vi "MagX Probes to Listbox.vi"(8 "error in":errorcluster, 10 "Probes":T1[](array[typedef]), 11 "Listbox ref":refnum<vi>) -> (0 "error out":errorcluster, 3 "Listbox ref out":refnum<vi>)   [LabVIEW 2024]
uses:
  Probe info.ctl
panel:
  out "Listbox out":i32(listbox)
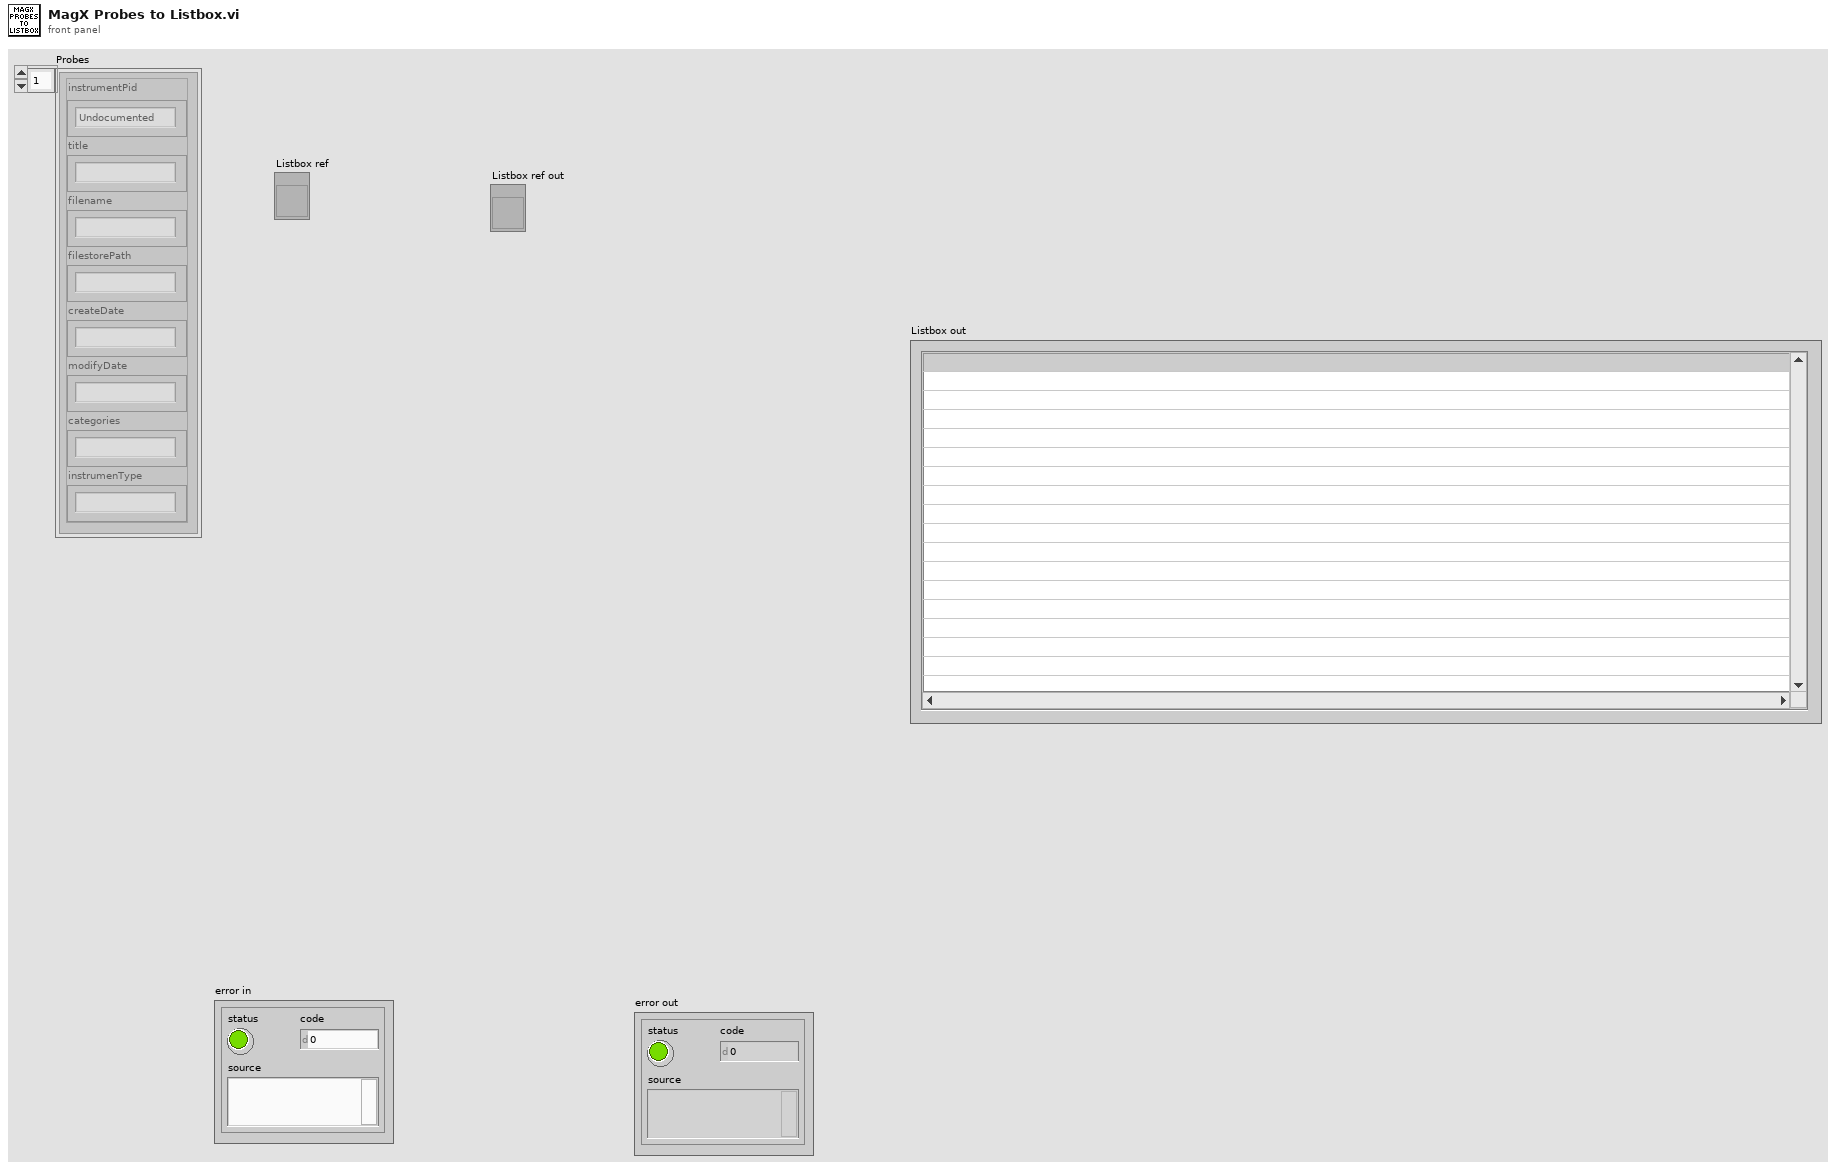
[diagram p1: front panel]
types:
  T1 = typedef "Probe info.ctl" = cluster{"instrumentPid":string, "title":string, "filename":string, "filestorePath":string, "createDate":string, "modifyDate":string, "categories":string, "instrumenType":string}
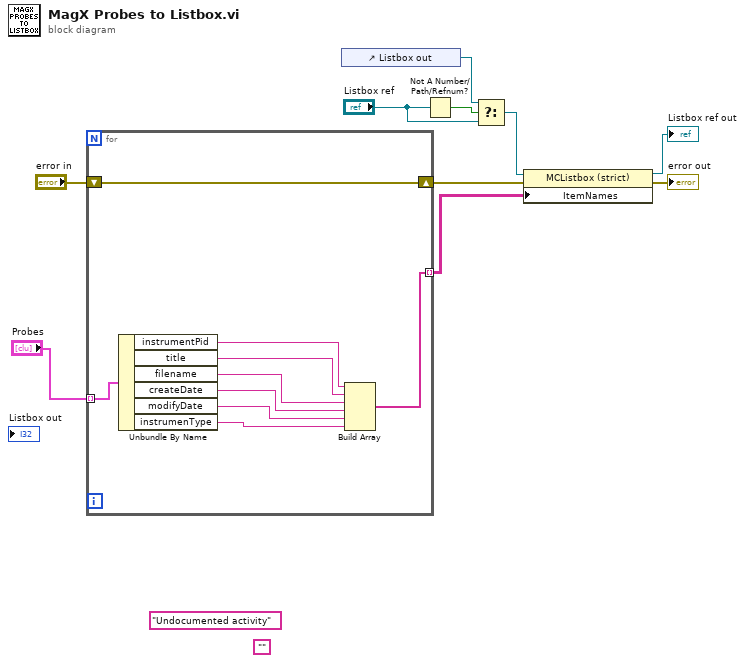
[diagram p0: block diagram]
diagram:
  (unwired) ""
  (unwired) "Undocumented activity"
  n1 = for {
    shift-right: [w19] -> w7
    shift-left: "error in" -> [w19]
    tunnel: [w11] -> w6 mode=indexing
    tunnel: "Probes" -> [w18] mode=indexing
    n2 = Unbundle By Name(w18) -> ("instrumentPid"=w17:string, "title"=w16:string, "filename"=w15:string, "createDate"=w14:string, "modifyDate"=w13:string, "instrumenType"=w12:string)
    n3 = Build Array(w17, w16, w15, w14, w13, w12) -> (w11:string[])
  }
  n4 = control-ref of="Listbox out"() -> (w4:refnum<vi>)
  n5 = Not A Number/Path/Refnum?(number/path/refnum="Listbox ref") -> (NaN/Path/Refnum?=w5:bool)
  n6 = Select(t=w4, s=w5, f="Listbox ref") -> (s? t:f=w2:refnum<vi>)
  n7 = property class="MCListbox (strict)"(reference=w2, error in=w7, "ItemNames"=w6) -> (reference out=→"Listbox ref out":refnum<vi>, error out=→"error out":errorcluster)
